vi "ParameterAT1.vi"(8 "error in (no error)":errorcluster, 9 "Integ Time (0: Short)":enum16{"SHORT", "MED/LONG"}(ring), 10 "Voltage Level (1.0)":dbl=1.0 min=0.005 max=20.0 format="%.3f", 11 "VISA resource name":refnum<visa-resource-name>) -> (0 "error out":errorcluster, 2 "Parameter At1":dbl format="%.3f", 3 "VISA resource name out":refnum<visa-resource-name>)   [LabVIEW 2015, in "Agilent 428X Series.lvlib"]
doc: "This panel is to calculate the parameter of AT1.\n\nDisclaimer: All accuracy calculation VI's are not part of the original \n driver. They are provided for supplementry purpose only.\n If user desires very high accuracy data, please do or \n check the calculation seperately."
uses:
  <instrlib>/Agilent 428X Series/Agilent 428X Series.lvlib
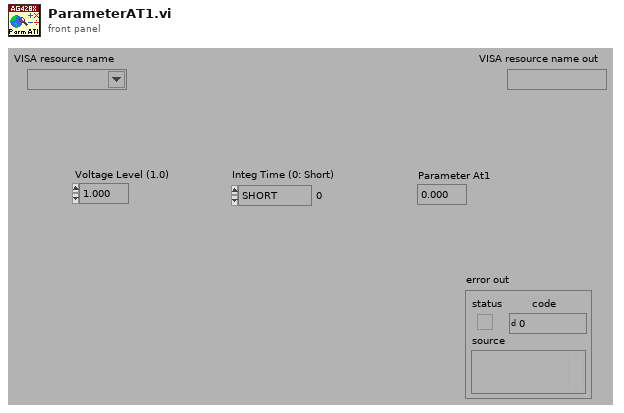
[diagram p1: front panel]
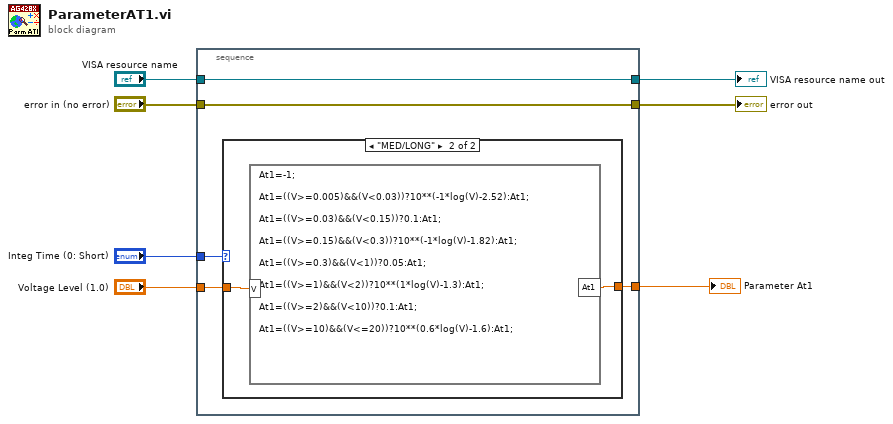
[diagram p0: block diagram]
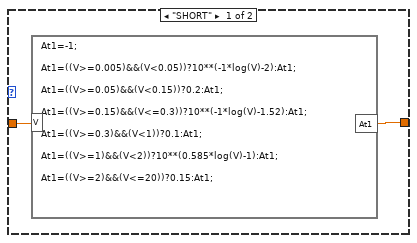
[diagram p2: hidden frame]
diagram:
  n1 = stacked-sequence {
    tunnel: [w12] -> w6
    tunnel: "Voltage Level (1.0)" -> [w11]
    tunnel: "error in (no error)" -> [w9]
    tunnel: "VISA resource name" -> [w10]
    tunnel: [w10] -> w3
    tunnel: [w9] -> w2
    tunnel: "Integ Time (0: Short)" -> [w8]
    frame #0 {
      n2 = case shown="\"MED/LONG\"" w8 {
        tunnel: w11 -> [w13 w16]
        tunnel: [w14 w15] -> w12
        frame "SHORT" {
          n3 = formula code="At1=-1;\n\nAt1=((V>=0.005)&&(V<0.05))?10**(-1*log(V)-2):At1;\n\nAt1=((V>=0.05)&&(V<0.15))?0.2:At1;\n\nAt1=((V>=0.15)&&(V<=0.3))?10**(-1*log(V)-1.52):At1;\n\nAt1=((V>=0.3)&&(V<1))?0.1:At1;\n\nAt1=((V>=1)&&(V<2))?10**(0.585*log(V)-1):At1;\n\nAt1=((V>=2)&&(V<=20))?0.15:At1;"("V"=w13) -> ("At1"=w14:dbl)
        }
        frame "MED/LONG" {
          n4 = formula code="At1=-1;\n\nAt1=((V>=0.005)&&(V<0.03))?10**(-1*log(V)-2.52):At1;\n\nAt1=((V>=0.03)&&(V<0.15))?0.1:At1;\n\nAt1=((V>=0.15)&&(V<0.3))?10**(-1*log(V)-1.82):At1;\n\nAt1=((V>=0.3)&&(V<1))?0.05:At1;\n\nAt1=((V>=1)&&(V<2))?10**(1*log(V)-1.3):At1;\n\nAt1=((V>=2)&&(V<10))?0.1:At1;\n\nAt1=((V>=10)&&(V<=20))?10**(0.6*log(V)-1.6):At1;"("V"=w16) -> ("At1"=w15:dbl)
        }
      }
    }
  }
  "error out" <- w2
  "VISA resource name out" <- w3
  "Parameter At1" <- w6
